vi "AllowEdgeStartCheck.vi"(0 "reference in":refnum<class "ClassDiagramGraph.lvclass">, 1 "EdgeStartNode":refnum<class "AbstractNode.lvclass">, 2 "GraphButton":u32, 5 "error in (no error)":errorcluster) -> (14 "reference out":refnum<class "ClassDiagramGraph.lvclass">, 16 "Allowed":bool, 19 "error out":errorcluster)   [LabVIEW 2014, in "ClassDiagramGraph.lvclass"]
uses:
  <resource>/Framework/Providers/Open_GDS/UML/ClassDiagramGraph_class/ClassDiagramGraph.lvclass
  <resource>/Framework/Providers/Open_GDS/UML/AbstractNode_class/AbstractNode.lvclass
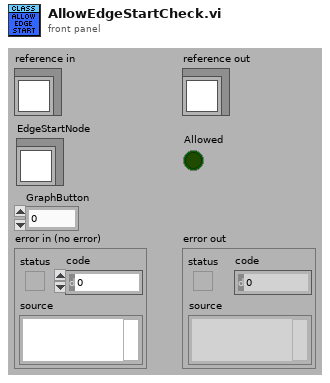
[diagram p1: front panel]
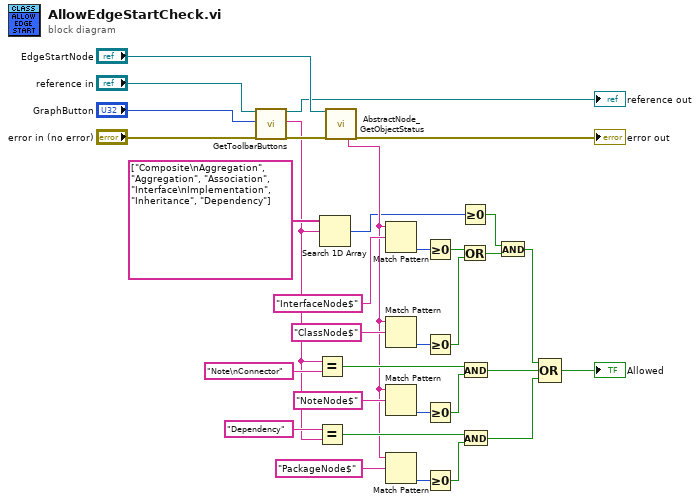
[diagram p0: block diagram]
diagram:
  n1 = call-dynamic "GetToolbarButtons.vi"("reference in"="reference in", "GraphButton"="GraphButton", "error in (no error)"="error in (no error)") -> ("reference out"=→"reference out":refnum<class "ClassDiagramGraph.lvclass">, "Text"=w3:string, "error out"=w26:errorcluster)  [unwired: 12 in, 2 out]
  n2 = Equal?(x=w3, y="Note\nConnector" ("Text")) -> (x = y?=w16:bool)
  n3 = Equal?(x="Dependency" ("Text"), y=w3) -> (x = y?=w11:bool)
  n4 = Search 1D Array(1D array=string[] ["Composite\nAggregation", "Aggregation", "Association", "Interface\nImplementation", "Inheritance", "Dependency"], element=w3) -> (index of element=w2:i32)  [unwired: 1 in]
  n5 = call <resource>:"AbstractNode_GetObjectStatus.vi"("reference in"="EdgeStartNode", "error in (no error)"=w26) -> ("Class name"=w8:string, "error out"=→"error out":errorcluster)  [unwired: 16 out]
  n6 = Match Pattern(string=w8, regular expression="InterfaceNode$") -> (offset past match=w21:i32)  [unwired: 4 out]
  n7 = Match Pattern(string=w8, regular expression="ClassNode$") -> (offset past match=w20:i32)  [unwired: 4 out]
  n8 = Match Pattern(string=w8, regular expression="NoteNode$") -> (offset past match=w22:i32)  [unwired: 4 out]
  n9 = Match Pattern(string=w8, regular expression="PackageNode$") -> (offset past match=w10:i32)  [unwired: 4 out]
  n10 = Greater Or Equal To 0?(x=w21) -> (x >= 0?=w19:bool)
  n11 = Greater Or Equal To 0?(x=w20) -> (x >= 0?=w18:bool)
  n12 = Greater Or Equal To 0?(x=w22) -> (x >= 0?=w15:bool)
  n13 = Greater Or Equal To 0?(x=w10) -> (x >= 0?=w7:bool)
  n14 = Greater Or Equal To 0?(x=w2) -> (x >= 0?=w1:bool)
  n15 = Or(x=w19, y=w18) -> (x .or. y?=w17:bool)
  n16 = And(x=w16, y=w15) -> (x .and. y?=w13:bool)
  n17 = And(x=w11, y=w7) -> (x .and. y?=w12:bool)
  n18 = And(x=w1, y=w17) -> (x .and. y?=w14:bool)
  n19 = Compound Arithmetic op=OR(w14, w13, w12) -> (→"Allowed":bool)
